vi "SORT POS.vi"(9 "$DirectionNum_":T2(ring), 10 "Array in":T3(array[cluster]), 11 "Image In":T1) -> (2 "Array out":T3(array[cluster]))   [LabVIEW 2019]
uses:
  <vilib>/vision/Image Controls.llb/IMAQ Image.ctl
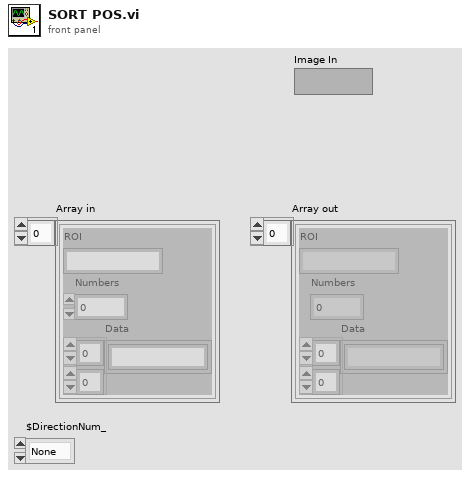
[diagram p1: front panel]
types:
  T1 = typedef "IMAQ Image.ctl" = refnum<image>
  T2 = enum16{"None", "Image左上", "Image左下", "Image右上", "Image右下"}
  T3 = cluster{"ROI":string, "Numbers":i32, "Data":string[][]}[]
  T4 = cluster{"ROI":string, "Numbers":i32, "Data":string[][]}
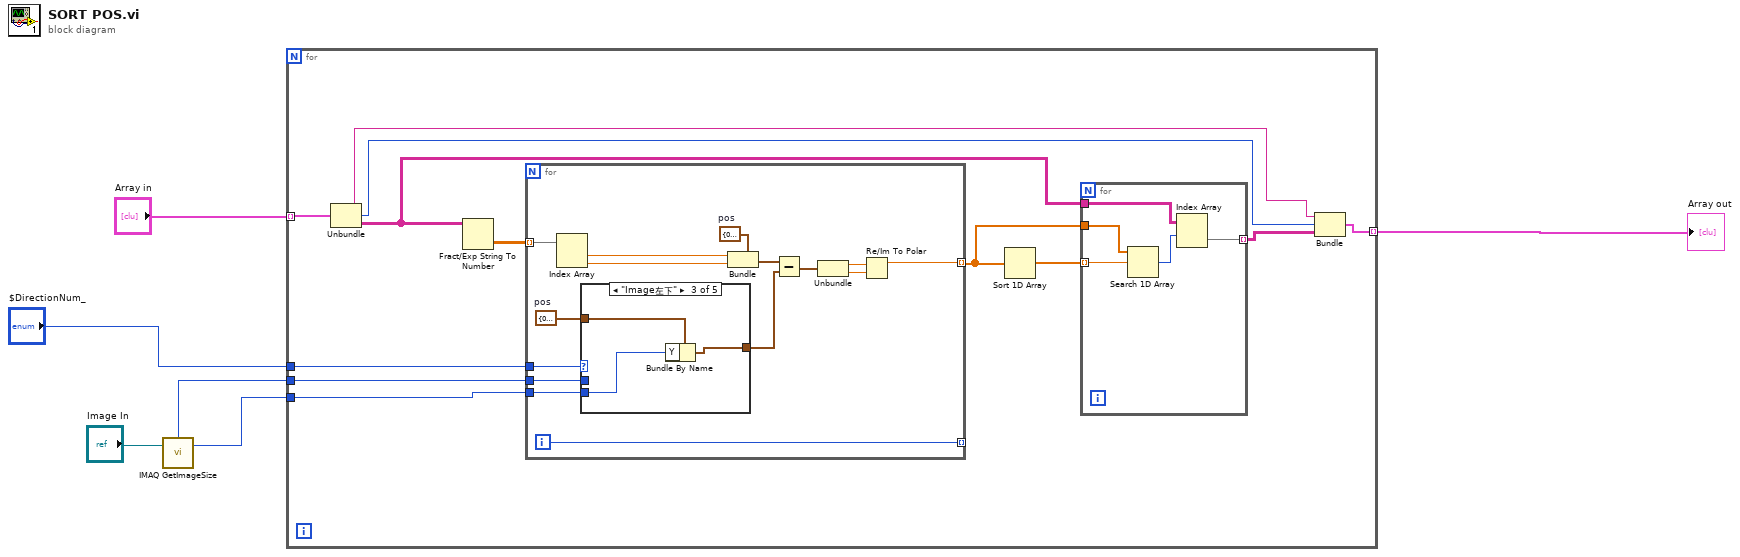
[diagram p0: block diagram]
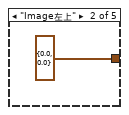
[diagram p3: hidden frame]
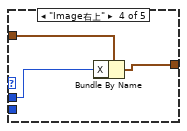
[diagram p4: hidden frame]
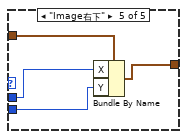
[diagram p5: hidden frame]
diagram:
  n1 = call "IMAQ GetImageSize"("Image"="Image In") -> ("Y Resolution"=w3:i32, "X Resolution"=w2:i32)  [unwired: 3 in, 1 out]
  n2 = for {
    tunnel: "Array in" -> [w17] mode=indexing
    tunnel: "$DirectionNum_" -> [w18]
    tunnel: w3 -> [w15]
    tunnel: w2 -> [w14]
    tunnel: [w7] -> w1 mode=indexing
    n3 = Unbundle(w17) -> ("ROI"=w8:string, "Numbers"=w9:i32, "Data"=w11:string[][])
    n4 = Fract/Exp String To Number(string=w11) -> (number=w16:dbl[][])  [unwired: 3 in, 1 out]
    n5 = for {
      tunnel: w18 -> [w38]
      tunnel: w16 -> [w37] mode=indexing
      tunnel: w15 -> [w30]
      tunnel: w14 -> [w29]
      tunnel: [w25] -> w13 mode=indexing
      tunnel: [w24] -> _ mode=indexing
      i -> [w24]
      w31 = cluster{"X":dbl, "Y":dbl} {"X"=0.0, "Y"=0.0}  # pos
      w32 = cluster{"X":dbl, "Y":dbl} {"X"=0.0, "Y"=0.0}  # pos
      n6 = Index Array(array=w37) -> (element #1=w36:dbl, element #2=w35:dbl)  [unwired: 2 in]
      n7 = case shown="\"Image左下\"" w38 {
        tunnel: [w39 cluster{dbl, dbl} {0.0, 0.0} ("y") w42 w45 w49] -> w33
        tunnel: w31 -> [w39 _ w43 w46 w50]
        tunnel: w30 -> [_ _ w41 _ w47]
        tunnel: w29 -> [_ _ _ w44 w48]
        frame "None", Default {
        }
        frame "Image左上" {
        }
        frame "Image左下" {
          n8 = Bundle By Name(cluster=w43, "Y"=w41) -> (w42:cluster{"X":dbl, "Y":dbl})
        }
        frame "Image右上" {
          n9 = Bundle By Name(cluster=w46, "X"=w44) -> (w45:cluster{"X":dbl, "Y":dbl})
        }
        frame "Image右下" {
          n10 = Bundle By Name(cluster=w50, "X"=w48, "Y"=w47) -> (w49:cluster{"X":dbl, "Y":dbl})
        }
      }
      n11 = Bundle(cluster=w32, "X"=w36, "Y"=w35) -> (w34:cluster{"X":dbl, "Y":dbl})
      n12 = Subtract(x=w34, y=w33) -> (x-y=w28:cluster{"X":dbl, "Y":dbl})
      n13 = Unbundle(w28) -> ("X"=w26:dbl, "Y"=w27:dbl)
      n14 = Re/Im To Polar(2:w27, 3:w26) -> (1:w25:dbl)  [unwired: 1 out]
    }
    n15 = Sort 1D Array(array=w13) -> (sorted array=w12:dbl[])
    n16 = for {
      tunnel: w13 -> [w23]
      tunnel: w12 -> [w22] mode=indexing
      tunnel: w11 -> [w21]
      tunnel: [w19] -> w10 mode=indexing
      n17 = Search 1D Array(1D array=w23, element=w22) -> (index of element=w20:i32)  [unwired: 1 in]
      n18 = Index Array(array=w21, index (row)=w20) -> (element=w19:string[])  [unwired: 1 in]
    }
    n19 = Bundle("ROI"=w8, "Numbers"=w9, "Data"=w10) -> (w7:T4)  [unwired: 1 in]
  }
  "Array out" <- w1
